vi "Calculate Intersection.vi"(10 "Rectangle 2":T1, 11 "Rectangle":T1) -> (2 "Intersection found":bool, 3 "Intersected Rectangle":T1)   [LabVIEW 2012]
doc: "Calculates the center of a rectangle"
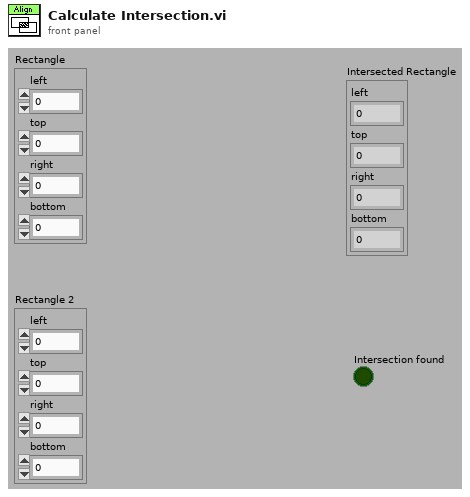
[diagram p1: front panel]
types:
  T1 = cluster{"left":i16, "top":i16, "right":i16, "bottom":i16}
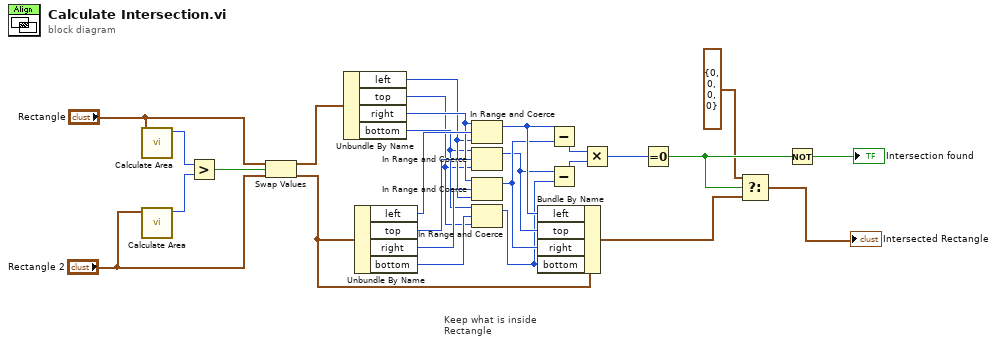
[diagram p0: block diagram]
diagram:
  # "Keep what is inside\nRectangle"
  n1 = call "Calculate Area.vi"("Rectangle"="Rectangle") -> ("Area"=w7:i32)  [unwired: 10 out]
  n2 = call "Calculate Area.vi"("Rectangle"="Rectangle 2") -> ("Area"=w6:i32)  [unwired: 10 out]
  n3 = Greater?(x=w7, y=w6) -> (0:w1:bool)
  n4 = Swap Values(12:"Rectangle", 13:w1, 14:"Rectangle 2") -> (1:w3:T1, 3:w2:T1)
  n5 = Unbundle By Name(w3) -> ("left"=w22:i16, "top"=w20:i16, "right"=w23:i16, "bottom"=w21:i16)
  n6 = Unbundle By Name(w2) -> ("left"=w27:i16, "top"=w24:i16, "right"=w25:i16, "bottom"=w26:i16)
  n7 = In Range and Coerce(upper limit=w23, x=w27, lower limit=w22) -> (coerced(x)=w19:i16)  [unwired: 1 out]
  n8 = In Range and Coerce(upper limit=w21, x=w24, lower limit=w20) -> (coerced(x)=w17:i16)  [unwired: 1 out]
  n9 = In Range and Coerce(upper limit=w23, x=w25, lower limit=w22) -> (coerced(x)=w18:i16)  [unwired: 1 out]
  n10 = In Range and Coerce(upper limit=w21, x=w26, lower limit=w20) -> (coerced(x)=w16:i16)  [unwired: 1 out]
  n11 = Bundle By Name(cluster=w2, "left"=w19, "top"=w17, "right"=w18, "bottom"=w16) -> (w11:T1)
  n12 = Subtract(x=w19, y=w18) -> (x-y=w15:i16)
  n13 = Subtract(x=w17, y=w16) -> (x-y=w14:i16)
  n14 = Multiply(x=w15, y=w14) -> (x*y=w13:i16)
  n15 = Equal To 0?(x=w13) -> (x = 0?=w12:bool)
  n16 = Select(t=T1 {"left"=0, "top"=0, "right"=0, "bottom"=0}, s=w12, f=w11) -> (s? t:f=→"Intersected Rectangle":T1)
  n17 = Not(x=w12) -> (.not. x?=→"Intersection found":bool)
